vi "DSF.Engine.Transfer Group.Increment Iteration.vi"(8 "error in (no error)":errorcluster, 11 "Transfer Group in":refnum<class "DSF.Engine.Transfer Group.lvclass">) -> (0 "error out":errorcluster, 3 "Transfer Group out":refnum<class "DSF.Engine.Transfer Group.lvclass">)   [LabVIEW 2017, in "Data Sharing Framework Engine.lvlib" / "DSF.Engine.Transfer Group.lvclass"]
uses:
  DSF.Engine.Transfer Group.lvclass
  DSF.Engine.Transfer Group.lvclass/DSF.Engine.Transfer Group.ctl
  Source/Data Sharing Framework Core/Engine/Timing/Engine Timing.lvclass/Engine Timing.ctl
  Source/Data Sharing Framework Core/Engine/Timing/Engine Timing.lvclass
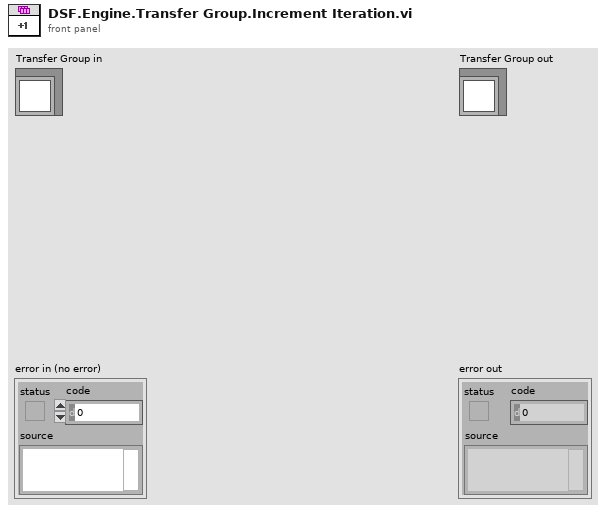
[diagram p1: front panel]
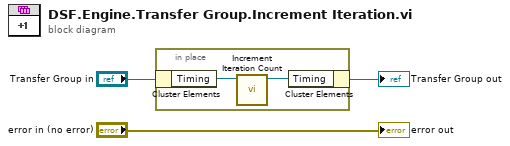
[diagram p0: block diagram]
diagram:
  n1 = in-place {
    n2 = in-place-cluster #1("Transfer Group in") -> ("Timing"=w5:refnum<class "Engine Timing.lvclass">)
    n3 = call "Increment Iteration Count.vi"("Timing in"=w5) -> ("Timing out"=w4:refnum<class "Engine Timing.lvclass">)  [unwired: 10 in]
    n4 = in-place-cluster #1("Timing"=w4) -> (→"Transfer Group out":refnum<class "DSF.Engine.Transfer Group.lvclass">)
  }
  "error out" <- "error in (no error)"
